vi "load.vi"(8 "error in (no error)":errorcluster, 10 "XML String":string, 11 "RoiGeneric in":refnum<class "RoiGeneric.lvclass">) -> (0 "error out":errorcluster, 3 "RoiGeneric out":refnum<class "RoiGeneric.lvclass">)   [LabVIEW 2010, in "RoiGeneric.lvclass"]
uses:
  RoiGeneric.lvclass
  xml_cluster.ctl
  attributes_cluster.ctl
  space_vector_cluster.ctl
  RoiGeneric.lvclass/RoiGeneric.ctl
  common/classes/SpaceVector/SpaceVector/SpaceVector.lvclass
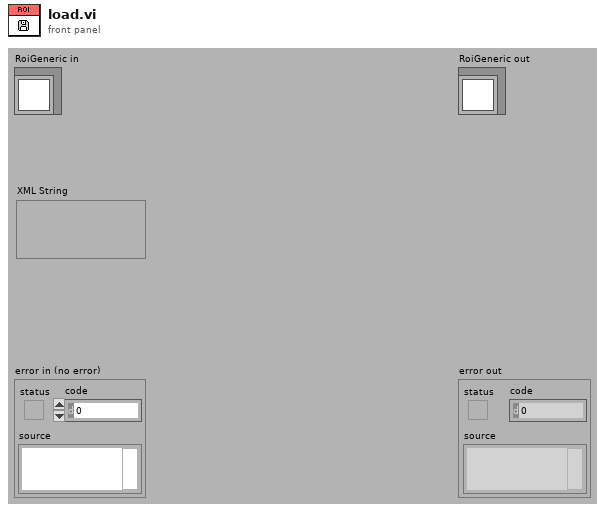
[diagram p1: front panel]
types:
  T1 = typedef "RoiGeneric.lvclass/xml_cluster.ctl" = cluster{"#attributes":T2, "center":T3, "dimensions":T3}
  T2 = typedef "RoiGeneric.lvclass/attributes_cluster.ctl" = cluster{"type":string, "ID":string}
  T3 = typedef "RoiGeneric.lvclass/space_vector_cluster.ctl" = cluster{"x":dbl[unit], "y":dbl[unit], "z":dbl[unit]}
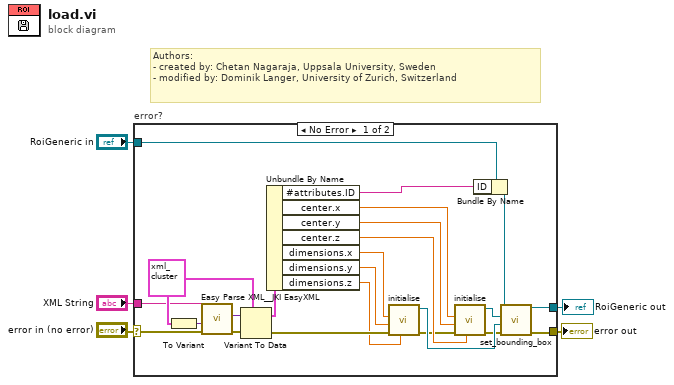
[diagram p0: block diagram]
diagram:
  # "Authors: \n- created by: Chetan Nagaraja, Uppsala University, Sweden\n- modified by: Dominik Langer, University of Zurich, Switzerland"
  n1 = case "error?" shown="No Error" "error in (no error)" {
    selector: "error in (no error)" -> [w10 w30]
    tunnel: [w17 w30] -> w4
    tunnel: [w16 w29] -> w2
    tunnel: "RoiGeneric in" -> [w8 w29]
    tunnel: "XML String" -> [w9 _]
    frame No Error {
      w11 = T1 {"#attributes"={"type"="ROI", "ID"=""}, "center"={"x"=0.0, "y"=0.0, "z"=0.0}, "dimensions"={"x"=0.0, "y"=0.0, "z"=0.0}} ("RoiGeneric")
      n2 = To Variant(anything=w11) -> (Variant=w25:variant)
      n3 = call <vilib>:"Easy Parse XML__JKI EasyXML.vi"("error in (no error)"=w10, "LabVIEW Data (Type)"=w25, "XML String"=w9) -> ("error out"=w26:errorcluster, "LabVIEW Data"=w27:variant)  [unwired: 7 in]
      n4 = Variant To Data(error in=w26, Variant=w27, type=w11) -> (error out=w21:errorcluster, data=w28:T1)
      n5 = Unbundle By Name(w28) -> ("#attributes.ID"=w6:string, "center.x"=w24:dbl[unit], "center.y"=w23:dbl[unit], "center.z"=w22:dbl[unit], "dimensions.x"=w20:dbl[unit], "dimensions.y"=w19:dbl[unit], "dimensions.z"=w18:dbl[unit])
      n6 = call "initialise.vi"("z"=w18, "error in (no error)"=w21, "y"=w19, "x"=w20) -> ("error out"=w12:errorcluster, "SpaceVector out"=w15:refnum<class "SpaceVector.lvclass">)  [unwired: 6 in]
      n7 = call "initialise.vi"("z"=w22, "error in (no error)"=w12, "y"=w23, "x"=w24) -> ("error out"=w13:errorcluster, "SpaceVector out"=w14:refnum<class "SpaceVector.lvclass">)  [unwired: 6 in]
      n8 = Bundle By Name(cluster=w8, "ID"=w6) -> (w7:refnum<class "RoiGeneric.lvclass">)
      n9 = call-dynamic "set_bounding_box.vi"("error in (no error)"=w13, "new size"=w15, "new center"=w14, "RoiGeneric in"=w7) -> ("error out"=w17:errorcluster, "RoiGeneric out"=w16:refnum<class "RoiGeneric.lvclass">)  [unwired: 6 in]
    }
    frame Error {
    }
  }
  "error out" <- w4
  "RoiGeneric out" <- w2
